vi "colorProcessing.vi"(4 "LED Color":T4={"Hue"={107.81818389892578, 139.81818389892578}, "Sat"={176.07142857142858, 255.0}, "Val"={40.53571428571429, 255.0}} {"Hue" scale=0.0..255.0 scale format="%#_3g"}, 6 "Color Mode":u16(ring)=3 items=["RGB", "HSL", "HSV", "HSI"], 7 "Source":enum32{"Files", "Camera"}(tab), 8 "Camera Type":T1=enum."MS HD3000 square", 11 "camImage":T3) -> (3 "Results":T2 {"Score" format="%#_3g"; "Pixels"."Rectangle"."bottomY" format="%#_3g"; "Pixels"."Rectangle"."rightX" format="%#_3g"; "Pixels"."Rectangle"."topY" format="%#_3g"; "Pixels"."Rectangle"."leftX" format="%#_3g"; "Normalized"."Rectangle"."bottomY" format="%#_2g"; "Normalized"."Rectangle"."rightX" format="%#_2g"; "Normalized"."Rectangle"."topY" format="%#_2g"; "Normalized"."Rectangle"."leftX" format="%#_2g"; "Normalized"."Center"."?" format="%#_3g"; "Normalized"."Center"."?" format="%#_3g"; "Distance (ft)" format="%#_3g"})   [LabVIEW 2016]
uses:
  Vision Support Code/Camera Types.ctl
  <vilib>/vision/Image Controls.llb/IMAQ Image.ctl
  <vilib>/vision/NI_Vision_Development_Module.lvlib
panel:
  in  "Line Border":cluster{"Top":dbl, "Bottom":dbl}={"Top"=6.0, "Bottom"=1.0}
  in  "Use Calibration":bool=TRUE
  out "Instructions:":string="Use Source to load image files from a directory, or use a USB or IP camera connected to your laptop. Use Camera Settings 1 and 2 to achieve a dark image with bright and colorful stripes.\nLED Color can encoded as HSL or related color modes. Calibrate to the same color as the strips being reflected to the camera.\nClick and draw a line in Original Image to auto-calibrate the LED Color. You may want to widen and tweak Sat and Val by hand.\nThe Annotate button affects drawing a rectangle around the stripes and labeling it with a distance in ft. Distance relies on knowing the Camera Type and lens calibration (it looks up the lens view angle).\n\nAdjust Score Cutoff to make the code more or less picky. If the color is not very unique, you may need to increase the number of particles considered. The diagram uses a Size Limit to ignore colored things that are too small. You may need to adjust it if you are targetting from far away.\n\nResults give you the distance to the target, the center and box in a normalized (-1 to 1) and pixel coordinates.\n\nBe sure to read about setting camera exposure and brightness to help simplify your image and acquire color saturated images.\n\nThere are lots of comments on the diagram to explain the code."
  in  "Particles":dbl=5.0
  in  "Score Cutoff %":dbl=70.0
  in  "Std Devs for Calibration":cluster{"H":dbl, "S":dbl, "V":dbl}={"H"=4.0, "S"=6.0, "V"=6.0}
  in  "image files":string[](array[string])
  in  "Images":i32(listbox)
  in  "Annotate":bool=TRUE
  out "Qualified Particles":i32
  out "Mask":T3(plugin-control)
  out "Original Image":T3(plugin-control)
  # "Legend:\n    Rectangle\n       Green - Good target, distance ft\n       Red - Bad target\n    Orange Text - Score in %"
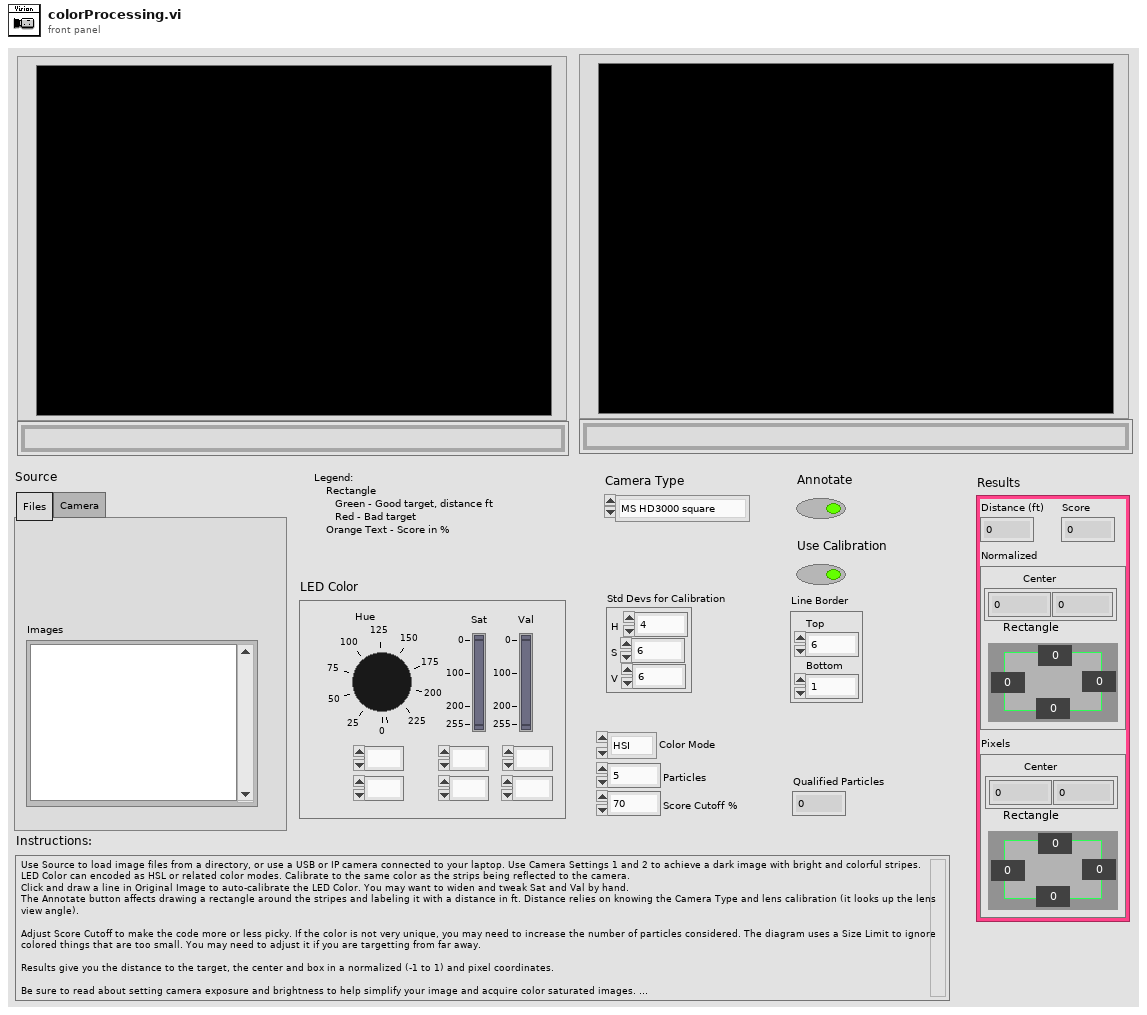
[diagram p1: front panel]
types:
  T1 = typedef "Camera Types.ctl" = enum16{"206", "1011", "1013", "MS HD3000 square", "MS HD3000 640x480"}
  T2 = cluster{"Distance (ft)":dbl, "Score":dbl, "Normalized":cluster{"Center":cluster{dbl, dbl}, "Rectangle":cluster{"leftX":dbl, "topY":dbl, "rightX":dbl, "bottomY":dbl}}, "Pixels":cluster{"Center":cluster{dbl, dbl}, "Rectangle":cluster{"leftX":dbl, "topY":dbl, "rightX":dbl, "bottomY":dbl}}}
  T3 = typedef "IMAQ Image.ctl" = refnum<image>
  T4 = cluster{"Hue":cluster{dbl, dbl}, "Sat":cluster{dbl, dbl}, "Val":cluster{dbl, dbl}}
  T5 = typedef "Image Type" = u32
  T6 = typedef "Particle Parameters" = i32
  T7 = cluster{cluster{dbl, dbl}, cluster{dbl, dbl}, cluster{dbl, dbl}}
  T8 = cluster{"Left":dbl, "Top":dbl, "Right":dbl, "Bottom":dbl}
  T9 = cluster{"Distance (ft)":dbl, "Score":dbl, "Normalized":cluster{"Center":cluster{dbl, dbl}, "Rectangle":cluster{"Numeric":dbl, "Numeric 2":dbl, "Numeric 3":dbl, "Numeric 5":dbl}}, "Pixels":cluster{"Center":cluster{dbl, dbl}, "Rectangle":cluster{"Numeric":dbl, "Numeric 2":dbl, "Numeric 3":dbl, "Numeric 5":dbl}}}
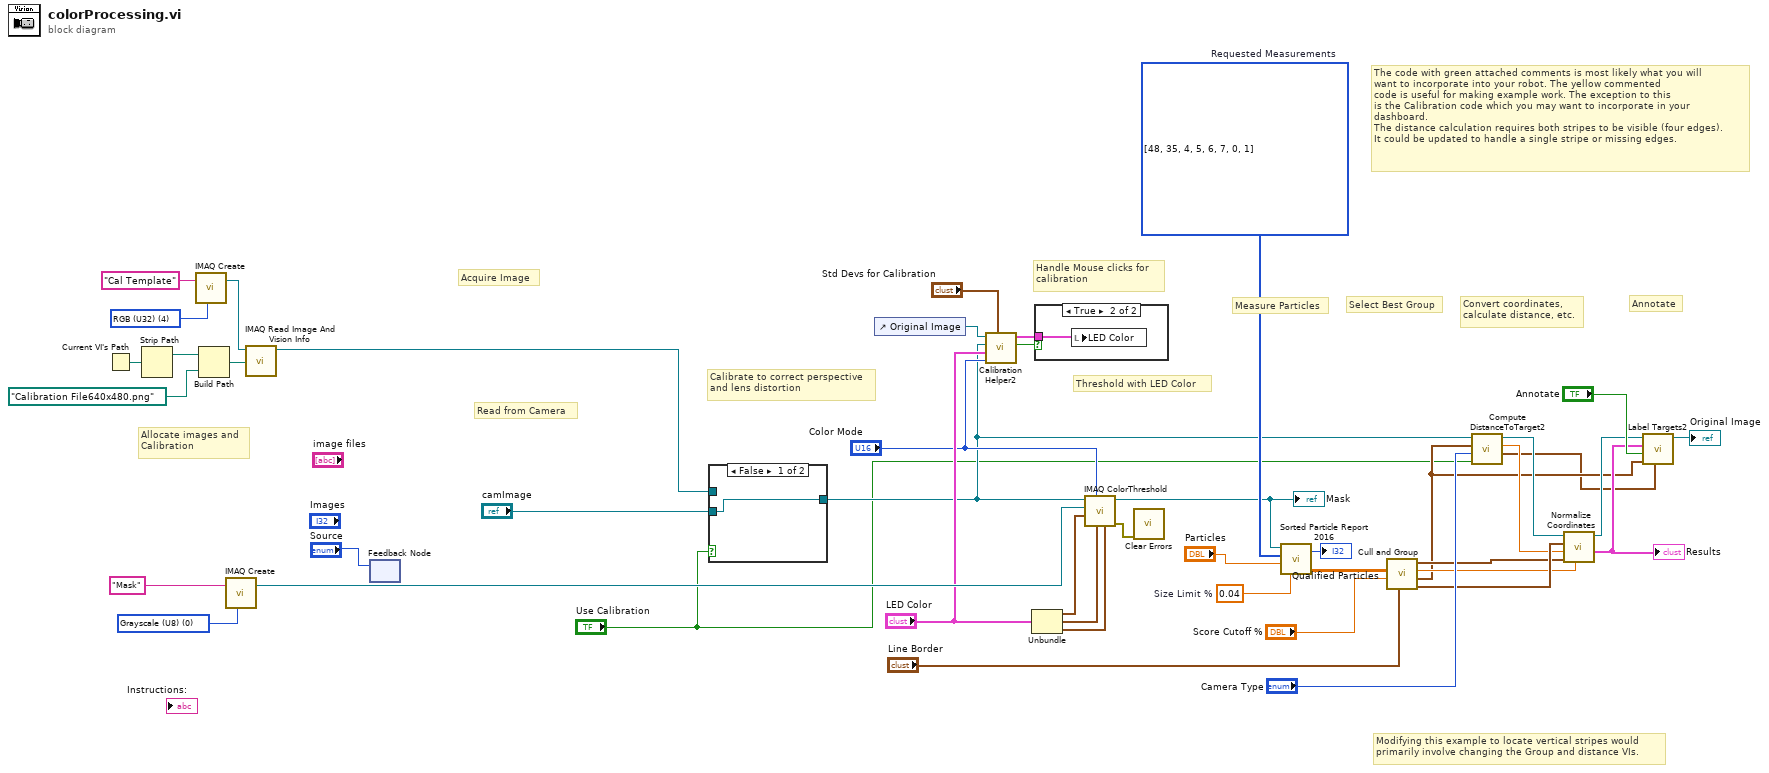
[diagram p0: block diagram]
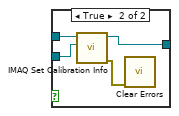
[diagram p2: hidden frame]
diagram:
  w29 = 0.04  # Size Limit %
  w41 = T5 4 items=["Grayscale (U8)", "Grayscale (I16)", "Grayscale (SGL)", "Complex (CSG)", "RGB (U32)", "HSL (U32)", "RGB (U64)", "Grayscale (U16)"] ("Image Type")
  w42 = T6[] [48, 35, 4, 5, 6, 7, 0, 1] items=["Center of Mass X", "Center of Mass Y", "First Pixel X", "First Pixel Y", "Bounding Rect Left", "Bounding Rect Top", "Bounding Rect Right", "Bounding Rect Bottom", "Max Feret Diameter Start X", "Max Feret Diameter Start Y", "Max Feret Diameter End X", "Max Feret Diameter End Y", "Max Horiz. Segment Length Left", "Max Horiz. Segment Length Right", "Max Horiz. Segment Length Row", "-", "Bounding Rect Width", "Bounding Rect Height", "Bounding Rect Diagonal", "Perimeter", "Convex Hull Perimeter", "Holes' Perimeter", "Max Feret Diameter", "Equivalent Ellipse Major Axis", "Equivalent Ellipse Minor Axis", "Equivalent Ellipse Minor Axis (Feret)", "Equivalent Rect Long Side", "Equivalent Rect Short Side", "Equivalent Rect Diagonal", "Equivalent Rect Short Side (Feret)", "Average Horiz. Segment Length", "Average Vert. Segment Length", "Hydraulic Radius", "Waddel Disk Diameter", "-", "Area", "Holes' Area", "Particle & Holes' Area", "Convex Hull Area", "Image Area", "-", "Number of Holes", "Number of Horiz. Segments", "Number of Vert. Segments", "-", "Orientation", "Max Feret Diameter Orientation", "-", "% Area/Image Area", "% Area/(Particle & Holes' Area)", "Ratio of Equivalent Ellipse Axes", "Ratio of Equivalent Rect Sides", "-", "Elongation Factor", "Compactness Factor", "Heywood Circularity Factor", "Type Factor", "-", "Sum X", "Sum Y", "Sum XX", "Sum XY", "Sum YY", "Sum XXX", "Sum XXY", "Sum XYY", "Sum YYY", "-", "Moment of Inertia XX", "Moment of Inertia XY", "Moment of Inertia YY", "Moment of Inertia XXX", "Moment of Inertia XXY", "Moment of Inertia XYY", "Moment of Inertia YYY", "Norm. Moment of Inertia XX", "Norm. Moment of Inertia XY", "Norm. Moment of Inertia YY", "Norm. Moment of Inertia XXX", "Norm. Moment of Inertia XXY", "Norm. Moment of Inertia XYY", "Norm. Moment of Inertia YYY", "Hu Moment 1", "Hu Moment 2", "Hu Moment 3", "Hu Moment 4", "Hu Moment 5", "Hu Moment 6", "Hu Moment 7"]  # Requested Measurements
  w45 = T5 0 items=["Grayscale (U8)", "Grayscale (I16)", "Grayscale (SGL)", "Complex (CSG)", "RGB (U32)", "HSL (U32)", "RGB (U64)", "Grayscale (U16)"] ("Image Type")
  # "Read from Camera"
  # "Calibrate to correct perspective\nand lens distortion"
  # "Handle Mouse clicks for\ncalibration"
  # "Measure Particles"
  # "Convert coordinates,\ncalculate distance, etc."
  # "Annotate"
  # "Select Best Group"
  # "Threshold with LED Color"
  # "Acquire Image"
  # "Modifying this example to locate vertical stripes would\nprimarily involve changing the Group and distance VIs."
  # "The code with green attached comments is most likely what you will\nwant to incorporate into your robot. The yellow commented\ncode is useful for making example work. The exception to this\nis the Calibration code which you may want to incorporate in your\ndashboard.\nThe distance calculation requires both stripes to be visible (four edges).\nIt could be updated to handle a single stripe or missing edges."
  # "Allocate images and\nCalibration"
  n1 = Current VI's Path() -> (path=w37:path)
  n2 = Strip Path(path=w37) -> (stripped path=w34:path)  [unwired: 1 out]
  n3 = call "IMAQ Create"("Image Name"="Cal Template", "Image Type"=w41) -> ("New Image"=w39:T3)  [unwired: 2 in, 2 out]
  n4 = Build Path(base path=w34, name or relative path=path "Calibration File640x480.png" ("Folder Location")) -> (appended path=w36:path)
  n5 = call "IMAQ Create"("Image Name"="Mask", "Image Type"=w45) -> ("New Image"=w43:T3)  [unwired: 2 in, 2 out]
  n6 = call "IMAQ Read Image And Vision Info"("File Path"=w36, "Image"=w39) -> ("Image Out"=w38:T3)  [unwired: 7 in, 2 out]
  n7 = feedback #1() -> ()  [unwired: 2 in]
  n8 = feedback-in #1("Source") -> ()
  n9 = case shown="False" "Use Calibration" {
    tunnel: [w46 w50] -> w4
    tunnel: w38 -> [_ w49]
    tunnel: "camImage" -> [w46 w47]
    frame False {
    }
    frame True {
      n10 = call "IMAQ Set Calibration Info"("Image Dst"=w47, "Image Src"=w49) -> ("error out"=w48:errorcluster, "Calibrated Image"=w50:T3)  [unwired: 8 in]
      n11 = call <vilib>:"Clear Errors.vi"("error in (no error)"=w48) -> ()  [unwired: 5 in, 2 out]
    }
  }
  n12 = control-ref of="Original Image"() -> (w25:refnum<vi>)
  n13 = call "Calibration Helper2.vi"("Std Devs"="Std Devs for Calibration", "Color Mode"="Color Mode", "Color Components"="LED Color", "Image"=w4, "Image Ctl Refnum"=w25) -> ("Changed"=w24:bool, "output color"=w23:T7)  [unwired: 5 in]
  n14 = Unbundle("LED Color") -> ("Hue"=w33:cluster{dbl, dbl}, "Sat"=w32:cluster{dbl, dbl}, "Val"=w31:cluster{dbl, dbl})
  n15 = case shown="True" w24 {
    tunnel: w23 -> [_ w51]
    frame False {
    }
    frame True {
      n16 = local write "LED Color"(w51) -> ()
    }
  }
  n17 = call "IMAQ ColorThreshold"("Blue or Luma or Val or Inten Range"=w31, "Green or Sat Range"=w32, "Color Mode"="Color Mode", "Red or Hue Range"=w33, "Image Dst"=w43, "Image Src"=w4) -> ("error out"=w26:errorcluster, "Image Dst Out"=w17:T3)  [unwired: 4 in]
  "Mask" <- w17
  n18 = call <vilib>:"Clear Errors.vi"("error in (no error)"=w26) -> ()  [unwired: 5 in, 2 out]
  n19 = call "Sorted Particle Report 2016.vi"("Min Area Size %"=w29, "Particle Count Limit"="Particles", "Pixel Measurements"=w42, "Image in"=w17) -> ("Sorted Data"=w19:dbl[][], "Particles"=→"Qualified Particles":i32)
  n20 = call "Cull and Group.vi"("Line Border"="Line Border", "Score Cutoff"="Score Cutoff %", "Sorted Data"=w19) -> ("Rect"=w15:T8, "Line"=w6:T8, "Score"=w9:dbl, "Center"=w11:cluster{"X":dbl, "Y":dbl})  [unwired: 5 in]
  n21 = call "Compute DistanceToTarget2.vi"("Calibrated"="Use Calibration", "Camera Type"="Camera Type", "Line"=w6, "Image Src"=w4) -> ("Edges"=w5:cluster{"X":sgl, "Y":sgl}[], "Distance (ft)"=w14:dbl, "Image Dst Out"=w13:T3)  [unwired: 5 in]
  n22 = call "Normalize Coordinates.vi"("Score"=w9, "Center"=w11, "Distance"=w14, "Bounding box"=w15, "Image in"=w13) -> ("Results"=w10:T9, "Image out"=w12:T3)  [unwired: 5 in]
  "Results" <- w10
  n23 = call "Label Targets2.vi"("Edges"=w5, "Line"=w6, "Annotate"="Annotate", "Results"=w10, "Image in"=w12) -> ("Image out"=→"Original Image":T3)  [unwired: 6 in]
